vi "Pre-Install Custom Action.vi"(10 "Variant":variant) -> (0 "error out":errorcluster)   [LabVIEW 2015]
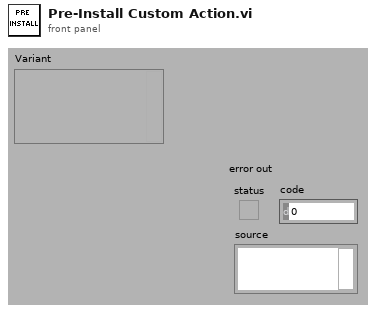
[diagram p1: front panel]
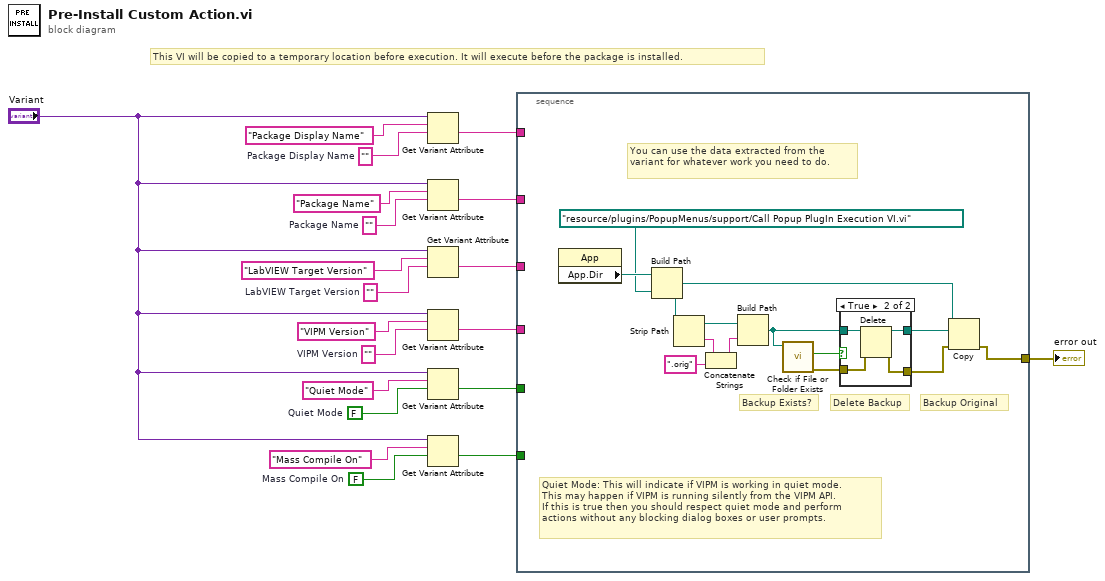
[diagram p0: block diagram]
diagram:
  w2 = FALSE  # Mass Compile On
  w4 = ""  # Package Display Name
  w11 = FALSE  # Quiet Mode
  w14 = ""  # VIPM Version
  w16 = ""  # LabVIEW Target Version
  w18 = ""  # Package Name
  # "This VI will be copied to a temporary location before execution. It will execute before the package is installed."
  n1 = Get Variant Attribute(Variant="Variant", name="Package Display Name", default value (empty Variant)=w4) -> (value=w10:string)  [unwired: 1 in, 3 out]
  n2 = Get Variant Attribute(Variant="Variant", name="Package Name", default value (empty Variant)=w18) -> (value=w9:string)  [unwired: 1 in, 3 out]
  n3 = Get Variant Attribute(Variant="Variant", name="LabVIEW Target Version", default value (empty Variant)=w16) -> (value=w8:string)  [unwired: 1 in, 3 out]
  n4 = Get Variant Attribute(Variant="Variant", name="VIPM Version", default value (empty Variant)=w14) -> (value=w7:string)  [unwired: 1 in, 3 out]
  n5 = Get Variant Attribute(Variant="Variant", name="Quiet Mode", default value (empty Variant)=w11) -> (value=w6:bool)  [unwired: 1 in, 3 out]
  n6 = Get Variant Attribute(Variant="Variant", name="Mass Compile On", default value (empty Variant)=w2) -> (value=w5:bool)  [unwired: 1 in, 3 out]
  n7 = stacked-sequence {
    tunnel: w10 -> [_]
    tunnel: w9 -> [_]
    tunnel: w8 -> [_]
    tunnel: w7 -> [_]
    tunnel: w6 -> [_]
    tunnel: w5 -> [_]
    tunnel: [w21] -> w1
    frame #0 {
      # "Backup Original"
      # "Delete Backup"
      # "Backup Exists?"
      # "Quiet Mode: This will indicate if VIPM is working in quiet mode.\nThis may happen if VIPM is running silently from the VIPM API.\nIf this is true then you should respect quiet mode and perform\nactions without any blocking dialog boxes or user prompts."
      # "You can use the data extracted from the variant for whatever work you need to do."
      n8 = property class="App"() -> ("App.Dir"=w33:path)  [unwired: 2 in, 2 out]
      n9 = Build Path(base path=w33, name or relative path=path "resource/plugins/PopupMenus/support/Call Popup PlugIn Execution VI.vi") -> (appended path=w31:path)
      n10 = Strip Path(path=w31) -> (stripped path=w30:path, name=w29:string)
      n11 = Concatenate Strings(w29, ".orig" ("string")) -> (w28:string)
      n12 = Build Path(base path=w30, name or relative path=w28) -> (appended path=w25:path)
      n13 = call <vilib>:"Check if File or Folder Exists.vi"("path"=w25) -> ("error out"=w23:errorcluster, "file or folder exists?"=w24:bool)  [unwired: 8 in, 1 out]
      n14 = case shown="True" w24 {
        tunnel: [w35 w39] -> w26
        tunnel: w25 -> [w35 w38]
        tunnel: w23 -> [w34 w37]
        tunnel: [w34 w36] -> w22
        frame False {
        }
        frame True {
          n15 = Delete(path (use dialog)=w38, error in=w37) -> (deleted path=w39:path, error out=w36:errorcluster)  [unwired: 3 in, 1 out]
        }
      }
      n16 = Copy(8:w22, 10:w26, 11:w31) -> (0:w21:errorcluster)  [unwired: 2 in, 2 out]
    }
  }
  "error out" <- w1
